vi "S4GUI_002.vi"(7 "Tab ObsEng":enum32{"Obs", "CCD modes", "Eng"}(tab)) -> ()   [LabVIEW 2018] (continued)
                n2194 = Flatten To String(anything=w4348, error in (no error)=w4351) -> (data string=w4353:string, error out=w4352:errorcluster)  [unwired: 2 in, 1 out]
                n2195 = call "Write flatted cluster.vi"("error in (no error)"=w4352, "flatted cluster"=w4353, "Interface in"=w4344) -> ("error out"=w4342:errorcluster, "Interface out"=w4343:refnum<class "Interface.lvclass">)  [unwired: 7 in]
                n2196 = call-dynamic "Write Interface.vi"("error in (no error)"=w4342, "Interface.lvclass"=w4343, "Channel in"=w4359) -> ("error out"=w4337:errorcluster, "Channel out"=w4336:refnum<class "Channel.lvclass">)  [unwired: 7 in]
                n2197 = call "Write section_name.vi"("error in (no error)"=w4337, "section_name"="CCD_ACS1", "Channel in"=w4336) -> ("error out"=w4338:errorcluster, "Channel out"=w4333:refnum<class "Channel.lvclass">)  [unwired: 7 in]
                n2198 = call-dynamic "save config.vi"("error in (no error)"=w4338, "file config"="lastsaved.cfg", "Channel in"=w4333) -> ("error out"=w4326:errorcluster, "Channel out"=w4327:refnum<class "Channel.lvclass">)  [unwired: 7 in]
                n2199 = call-dynamic "Read State Machine.vi"("error in (no error)"=w4326, "Device in"=w4327) -> ("error out"=w4341:errorcluster, "State Machine.lvclass"=w4331:refnum<class "State Machine.lvclass">, "Device out"=w4332:refnum<class "Channel.lvclass">)  [unwired: 7 in]
                n2200 = call-dynamic "Write State.vi"("error in (no error)"=w4341, "State"=60, "State Machine in"=w4331) -> ("error out"=w4340:errorcluster, "State Machine out"=w4330:refnum<class "State Machine.lvclass">)  [unwired: 7 in]
                n2201 = call-dynamic "Write State Machine.vi"("error in (no error)"=w4340, "State Machine.lvclass"=w4330, "Device in"=w4332) -> ("error out"=w4328:errorcluster, "Device out"=w4329:refnum<class "Channel.lvclass">)  [unwired: 7 in]
                n2202 = call-dynamic "Write Channel.vi"("error in (no error)"=w4328, "Channel.lvclass"=w4329, "Acquisition in"=w4358) -> ("error out"=w4355:errorcluster, "Acquisition out"=w4354:refnum<class "Acquisition.lvclass">)  [unwired: 7 in]
              }
            }
            n2203 = call-dynamic "Write AcquisitionA.vi"("error in (no error)"=w4164, "Acquisition.lvclass"=w4165, "S4ACS_GUI in"=w4166) -> ("error out"=w4172:errorcluster, "S4ACS_GUI out"=w4175:refnum<class "S4GUI.lvclass">)  [unwired: 7 in]
            n2204 = call "Write AcquisitionB.vi"("error in (no error)"=w4162, "Acquisition.lvclass"=w4163, "S4ACS_GUI in"=w4175) -> ("error out"=w4171:errorcluster, "S4ACS_GUI out"=w4174:refnum<class "S4GUI.lvclass">)  [unwired: 7 in]
            n2205 = call-dynamic "Write AcquisitionC.vi"("error in (no error)"=w4160, "Acquisition.lvclass"=w4161, "S4ACS_GUI in"=w4174) -> ("error out"=w4170:errorcluster, "S4ACS_GUI out"=w4173:refnum<class "S4GUI.lvclass">)  [unwired: 7 in]
            n2206 = call-dynamic "Write AcquisitionD.vi"("error in (no error)"=w4158, "Acquisition.lvclass"=w4159, "S4ACS_GUI in"=w4173) -> ("error out"=w4169:errorcluster, "S4ACS_GUI out"=w4168:refnum<class "S4GUI.lvclass">)  [unwired: 7 in]
            n2207 = Merge Errors(w4172, w4171, w4170, w4169) -> (w4167:errorcluster)
          }
        }
        n2208 = Concatenate Strings(w3924, " MODE SELECTED" ("User Event")) -> (w3929:string)
        n2209 = call-dynamic "Write sync.vi"("error in (no error)"=w3942, "sync"=w3944, "S4ACS_GUI in"=w3943) -> ("error out"=w3927:errorcluster, "S4ACS_GUI out"=w3928:refnum<class "S4GUI.lvclass">)  [unwired: 7 in]
        n2210 = call-dynamic "Write User Event.vi"("error in (no error)"=w3927, "User Event"=w3929, "S4GUI in"=w3928) -> ("error out"=w3925:errorcluster, "S4GUI out"=w3926:refnum<class "S4GUI.lvclass">)  [unwired: 7 in]
      }
      event "SendExpose": Value Change {
        n2211 = event-data() -> ("NewVal"=w4360:bool)  [unwired: 1 in]
        n2212 = disable-structure shown="Enabled" {
          disable-tunnel: w4360 -> [w4498 w4499]
          disable-tunnel: [w4497 w4499] -> w4361
          frame Disabled {
            n2213 = Not(x=w4498) -> (.not. x?=w4497:bool)
          }
          frame Enabled {
          }
        }
        n2214 = disable-structure shown="Enabled" {
          disable-tunnel: w4445 -> [w4460 w4496]
          disable-tunnel: w4444 -> [w4451 w4495]
          disable-tunnel: [w4448 w4496] -> w4363
          disable-tunnel: [w4447 w4495] -> w4362
          disable-tunnel: w4360 -> [w4446 _]
          frame Disabled {
            n2215 = call-dynamic "Read Sync Box.lvclass.vi"("error in (no error)"=w4451, "SPARC4_AC in"=w4460) -> ("error out"=w4453:errorcluster, "Sync Box.lvclass"=w4459:refnum<class "Sync Box.lvclass">, "SPARC4_AC out"=w4456:refnum<class "S4GUI.lvclass">)  [unwired: 7 in]
            n2216 = call-dynamic "Read Stream.vi"("error in (no error)"=w4453, "Server in"=w4459) -> ("error out"=w4452:errorcluster, "Stream.lvclass"=w4461:refnum<class "Stream.lvclass">, "Server out"=w4450:refnum<class "Sync Box.lvclass">)  [unwired: 7 in]
            n2217 = case shown="True" w4446 {
              tunnel: [w4464 w4481] -> w4454
              tunnel: w4461 -> [w4466 w4471]
              tunnel: [w4465 w4477] -> w4458
              tunnel: w4452 -> [w4463 w4469]
              tunnel: w4450 -> [w4462 w4470]
              tunnel: [w4462 w4470] -> w4449
              frame False {
                n2218 = call-dynamic "End.vi"("error in (no error)"=w4463, "Stream in"=w4466) -> ("error out"=w4464:errorcluster, "Stream out"=w4465:refnum<class "Stream.lvclass">)  [unwired: 8 in]
              }
              frame True {
                w4474 = errorcluster {"status"=FALSE, "code"=0, "source"=""} ("error in (no error)")
                w4492 = FALSE ("Wait Until Done")
                w4487 = FALSE ("Wait Until Done")
                n2219 = call-dynamic "Read comfile name1.vi"("error in (no error)"=w4469, "Stream in"=w4471) -> ("error out"=w4483:errorcluster, "comfile name1"=w4484:string, "Stream out"=w4480:refnum<class "Stream.lvclass">)  [unwired: 7 in]
                n2220 = call <vilib>:"Application Directory.vi"() -> ("Application Directory"=w4489:path)
                n2221 = call <vilib>:"Application Directory.vi"() -> ("Application Directory"=w4493:path)
                n2222 = Build Path(base path=w4493, name or relative path=w4484) -> (appended path=w4494:path)
                n2223 = Open VI Reference(vi path=w4494, error in (no error)=w4483) -> (vi reference=w4486:refnum<vi>, error out=w4485:errorcluster)  [unwired: 4 in]
                n2224 = invoke class="VI" method="Run VI"(reference=w4486, error in=w4485, "Wait until done"=w4487, "Auto Dispose Ref"=w4487) -> (reference out=w4476:refnum<vi>, error out=→"error out 7":errorcluster)  [unwired: 1 in, 3 out]
                n2225 = call-dynamic "Write commfile ref1.vi"("error in (no error)"=w4474, "commfile ref1"=w4476, "Stream in"=w4480) -> ("error out"=w4468:errorcluster, "Stream out"=w4479:refnum<class "Stream.lvclass">)  [unwired: 7 in]
                n2226 = call-dynamic "Read comfile name2.vi"("error in (no error)"=w4468, "Stream in"=w4479) -> ("error out"=w4467:errorcluster, "comfile name2"=w4482:string, "Stream out"=w4478:refnum<class "Stream.lvclass">)  [unwired: 7 in]
                n2227 = Build Path(base path=w4489, name or relative path=w4482) -> (appended path=w4488:path)
                n2228 = Open VI Reference(vi path=w4488, error in (no error)=w4467) -> (vi reference=w4490:refnum<vi>, error out=w4491:errorcluster)  [unwired: 4 in]
                n2229 = invoke class="VI" method="Run VI"(reference=w4490, error in=w4491, "Wait until done"=w4492, "Auto Dispose Ref"=w4492) -> (reference out=w4475:refnum<vi>, error out=→"error out 8":errorcluster)  [unwired: 1 in, 3 out]
                n2230 = call-dynamic "Write commfile ref2.vi"("error in (no error)"=w4474, "commfile ref2"=w4475, "Stream in"=w4478) -> ("error out"=w4481:errorcluster, "Stream out"=w4477:refnum<class "Stream.lvclass">)  [unwired: 7 in]
              }
            }
            n2231 = call-dynamic "Write Stream.vi"("error in (no error)"=w4454, "Stream.lvclass"=w4458, "Server in"=w4449) -> ("error out"=w4455:errorcluster, "Server out"=w4457:refnum<class "Sync Box.lvclass">)  [unwired: 7 in]
            n2232 = call-dynamic "Write Sync Box.lvclass.vi"("error in (no error)"=w4455, "Sync Box.lvclass"=w4457, "SPARC4_AC in"=w4456) -> ("error out"=w4447:errorcluster, "SPARC4_AC out"=w4448:refnum<class "S4GUI.lvclass">)  [unwired: 7 in]
          }
          frame Enabled {
          }
        }
        n2233 = call-dynamic "Read AcquisitionC.vi"("error in (no error)"=w4362, "S4ACS_GUI in"=w4363) -> ("error out"=w4387:errorcluster, "Acquisition.lvclass"=w4388:refnum<class "Acquisition.lvclass">)  [unwired: 7 in, 1 out]
        n2234 = call-dynamic "Read AcquisitionA.vi"("error in (no error)"=w4362, "S4ACS_GUI in"=w4363) -> ("error out"=w4424:errorcluster, "Acquisition.lvclass"=w4423:refnum<class "Acquisition.lvclass">, "S4ACS_GUI out"=w4440:refnum<class "S4GUI.lvclass">)  [unwired: 7 in]
        n2235 = call "Read AcquisitionB.vi"("error in (no error)"=w4362, "S4ACS_GUI in"=w4363) -> ("error out"=w4404:errorcluster, "Acquisition.lvclass"=w4405:refnum<class "Acquisition.lvclass">)  [unwired: 7 in, 1 out]
        n2236 = call-dynamic "Read AcquisitionD.vi"("error in (no error)"=w4362, "S4ACS_GUI in"=w4363) -> ("error out"=w4370:errorcluster, "Acquisition.lvclass"=w4371:refnum<class "Acquisition.lvclass">)  [unwired: 7 in, 1 out]
        n2237 = call-dynamic "Read Channel.vi"("error in (no error)"=w4370, "Acquisition in"=w4371) -> ("error out"=w4373:errorcluster, "Channel.lvclass"=w4375:refnum<class "Channel.lvclass">, "Acquisition out"=w4384:refnum<class "Acquisition.lvclass">)  [unwired: 7 in]
        n2238 = call-dynamic "Read Channel.vi"("error in (no error)"=w4387, "Acquisition in"=w4388) -> ("error out"=w4390:errorcluster, "Channel.lvclass"=w4392:refnum<class "Channel.lvclass">, "Acquisition out"=w4401:refnum<class "Acquisition.lvclass">)  [unwired: 7 in]
        n2239 = call-dynamic "Read Channel.vi"("error in (no error)"=w4404, "Acquisition in"=w4405) -> ("error out"=w4407:errorcluster, "Channel.lvclass"=w4409:refnum<class "Channel.lvclass">, "Acquisition out"=w4418:refnum<class "Acquisition.lvclass">)  [unwired: 7 in]
        n2240 = call-dynamic "Read Channel.vi"("error in (no error)"=w4424, "Acquisition in"=w4423) -> ("error out"=w4420:errorcluster, "Channel.lvclass"=w4422:refnum<class "Channel.lvclass">, "Acquisition out"=w4433:refnum<class "Acquisition.lvclass">)  [unwired: 7 in]
        n2241 = call-dynamic "Write wait_expose.vi"("error in (no error)"=w4373, "wait_expose"=w4361, "Channel in"=w4375) -> ("error out"=w4372:errorcluster, "Channel out"=w4374:refnum<class "Channel.lvclass">)  [unwired: 7 in]
        n2242 = call-dynamic "Write wait_expose.vi"("error in (no error)"=w4390, "wait_expose"=w4361, "Channel in"=w4392) -> ("error out"=w4389:errorcluster, "Channel out"=w4391:refnum<class "Channel.lvclass">)  [unwired: 7 in]
        n2243 = call-dynamic "Write wait_expose.vi"("error in (no error)"=w4407, "wait_expose"=w4361, "Channel in"=w4409) -> ("error out"=w4406:errorcluster, "Channel out"=w4408:refnum<class "Channel.lvclass">)  [unwired: 7 in]
        n2244 = call-dynamic "Write wait_expose.vi"("error in (no error)"=w4420, "wait_expose"=w4361, "Channel in"=w4422) -> ("error out"=w4419:errorcluster, "Channel out"=w4421:refnum<class "Channel.lvclass">)  [unwired: 7 in]
        n2245 = call-dynamic "Read State Machine.vi"("error in (no error)"=w4372, "Device in"=w4374) -> ("error out"=w4383:errorcluster, "State Machine.lvclass"=w4379:refnum<class "State Machine.lvclass">, "Device out"=w4380:refnum<class "Channel.lvclass">)  [unwired: 7 in]
        n2246 = call-dynamic "Read State Machine.vi"("error in (no error)"=w4389, "Device in"=w4391) -> ("error out"=w4400:errorcluster, "State Machine.lvclass"=w4396:refnum<class "State Machine.lvclass">, "Device out"=w4397:refnum<class "Channel.lvclass">)  [unwired: 7 in]
        n2247 = call-dynamic "Read State Machine.vi"("error in (no error)"=w4406, "Device in"=w4408) -> ("error out"=w4417:errorcluster, "State Machine.lvclass"=w4413:refnum<class "State Machine.lvclass">, "Device out"=w4414:refnum<class "Channel.lvclass">)  [unwired: 7 in]
        n2248 = call-dynamic "Read State Machine.vi"("error in (no error)"=w4419, "Device in"=w4421) -> ("error out"=w4432:errorcluster, "State Machine.lvclass"=w4428:refnum<class "State Machine.lvclass">, "Device out"=w4429:refnum<class "Channel.lvclass">)  [unwired: 7 in]
        n2249 = call-dynamic "Write State.vi"("error in (no error)"=w4383, "State"=40, "State Machine in"=w4379) -> ("error out"=w4382:errorcluster, "State Machine out"=w4378:refnum<class "State Machine.lvclass">)  [unwired: 7 in]
        n2250 = call-dynamic "Write State.vi"("error in (no error)"=w4400, "State"=40, "State Machine in"=w4396) -> ("error out"=w4399:errorcluster, "State Machine out"=w4395:refnum<class "State Machine.lvclass">)  [unwired: 7 in]
        n2251 = call-dynamic "Write State.vi"("error in (no error)"=w4417, "State"=40, "State Machine in"=w4413) -> ("error out"=w4416:errorcluster, "State Machine out"=w4412:refnum<class "State Machine.lvclass">)  [unwired: 7 in]
        n2252 = call-dynamic "Write State.vi"("error in (no error)"=w4432, "State"=40, "State Machine in"=w4428) -> ("error out"=w4431:errorcluster, "State Machine out"=w4427:refnum<class "State Machine.lvclass">)  [unwired: 7 in]
        n2253 = call-dynamic "Write State Machine.vi"("error in (no error)"=w4382, "State Machine.lvclass"=w4378, "Device in"=w4380) -> ("error out"=w4376:errorcluster, "Device out"=w4377:refnum<class "Channel.lvclass">)  [unwired: 7 in]
        n2254 = call-dynamic "Write State Machine.vi"("error in (no error)"=w4399, "State Machine.lvclass"=w4395, "Device in"=w4397) -> ("error out"=w4393:errorcluster, "Device out"=w4394:refnum<class "Channel.lvclass">)  [unwired: 7 in]
        n2255 = call-dynamic "Write State Machine.vi"("error in (no error)"=w4416, "State Machine.lvclass"=w4412, "Device in"=w4414) -> ("error out"=w4410:errorcluster, "Device out"=w4411:refnum<class "Channel.lvclass">)  [unwired: 7 in]
        n2256 = call-dynamic "Write State Machine.vi"("error in (no error)"=w4431, "State Machine.lvclass"=w4427, "Device in"=w4429) -> ("error out"=w4425:errorcluster, "Device out"=w4426:refnum<class "Channel.lvclass">)  [unwired: 7 in]
        n2257 = call-dynamic "Write Channel.vi"("error in (no error)"=w4376, "Channel.lvclass"=w4377, "Acquisition in"=w4384) -> ("error out"=w4368:errorcluster, "Acquisition out"=w4369:refnum<class "Acquisition.lvclass">)  [unwired: 7 in]
        n2258 = call-dynamic "Write Channel.vi"("error in (no error)"=w4393, "Channel.lvclass"=w4394, "Acquisition in"=w4401) -> ("error out"=w4386:errorcluster, "Acquisition out"=w4385:refnum<class "Acquisition.lvclass">)  [unwired: 7 in]
        n2259 = call-dynamic "Write Channel.vi"("error in (no error)"=w4410, "Channel.lvclass"=w4411, "Acquisition in"=w4418) -> ("error out"=w4403:errorcluster, "Acquisition out"=w4402:refnum<class "Acquisition.lvclass">)  [unwired: 7 in]
        n2260 = call-dynamic "Write Channel.vi"("error in (no error)"=w4425, "Channel.lvclass"=w4426, "Acquisition in"=w4433) -> ("error out"=w4438:errorcluster, "Acquisition out"=w4439:refnum<class "Acquisition.lvclass">)  [unwired: 7 in]
        n2261 = call-dynamic "Write AcquisitionA.vi"("error in (no error)"=w4438, "Acquisition.lvclass"=w4439, "S4ACS_GUI in"=w4440) -> ("error out"=w4437:errorcluster, "S4ACS_GUI out"=w4443:refnum<class "S4GUI.lvclass">)  [unwired: 7 in]
        n2262 = call "Write AcquisitionB.vi"("error in (no error)"=w4403, "Acquisition.lvclass"=w4402, "S4ACS_GUI in"=w4443) -> ("error out"=w4436:errorcluster, "S4ACS_GUI out"=w4442:refnum<class "S4GUI.lvclass">)  [unwired: 7 in]
        n2263 = call-dynamic "Write AcquisitionC.vi"("error in (no error)"=w4386, "Acquisition.lvclass"=w4385, "S4ACS_GUI in"=w4442) -> ("error out"=w4435:errorcluster, "S4ACS_GUI out"=w4441:refnum<class "S4GUI.lvclass">)  [unwired: 7 in]
        n2264 = call-dynamic "Write AcquisitionD.vi"("error in (no error)"=w4368, "Acquisition.lvclass"=w4369, "S4ACS_GUI in"=w4441) -> ("error out"=w4434:errorcluster, "S4ACS_GUI out"=w4367:refnum<class "S4GUI.lvclass">)  [unwired: 7 in]
        n2265 = Merge Errors(w4437, w4436, w4435, w4434) -> (w4366:errorcluster)
        n2266 = call-dynamic "Write mode EXPOSE.vi"("error in (no error)"=w4366, "mode EXPOSE"=w4361, "S4GUI in"=w4367) -> ("error out"=w4364:errorcluster, "S4GUI out"=w4365:refnum<class "S4GUI.lvclass">)  [unwired: 7 in]
      }
      event "CH1on": Value Change {
        n2267 = event-data() -> ("NewVal"=w4509:bool)  [unwired: 1 in]
        n2268 = call-dynamic "Read AcquisitionA.vi"("error in (no error)"=w4523, "S4ACS_GUI in"=w4524) -> ("error out"=w4515:errorcluster, "Acquisition.lvclass"=w4520:refnum<class "Acquisition.lvclass">, "S4ACS_GUI out"=w4516:refnum<class "S4GUI.lvclass">)  [unwired: 7 in]
        n2269 = call-dynamic "Read Channel.vi"("error in (no error)"=w4515, "Acquisition in"=w4520) -> ("error out"=w4514:errorcluster, "Channel.lvclass"=w4505:refnum<class "Channel.lvclass">, "Acquisition out"=w4519:refnum<class "Acquisition.lvclass">)  [unwired: 7 in]
        n2270 = call-dynamic "Read Stream.vi"("error in (no error)"=w4514, "Server in"=w4519) -> ("error out"=w4507:errorcluster, "Stream.lvclass"=w4508:refnum<class "Stream.lvclass">, "Server out"=w4506:refnum<class "Acquisition.lvclass">)  [unwired: 7 in]
        n2271 = case shown="False" w4509 {
          selector: w4509 -> [w4525 w4547]
          tunnel: [w4531 w4551] -> w4503
          tunnel: w4508 -> [w4540 _]
          tunnel: [w4539 w4554] -> w4502
          tunnel: w4507 -> [w4526 w4548]
          tunnel: w4506 -> [w4527 w4549]
          tunnel: [w4527 w4553] -> w4501
          tunnel: w4505 -> [w4538 w4550]
          tunnel: [w4536 w4550] -> w4500
          tunnel: [w4525 w4547] -> w4504
          frame False {
            # "força FALSE nos parametros do CCD"
            n2272 = call-dynamic "Read Interface.vi"("error in (no error)"=w4526, "Channel in"=w4538) -> ("error out"=w4535:errorcluster, "Interface.lvclass"=w4529:refnum<class "Interface.lvclass">, "Channel out"=w4537:refnum<class "Channel.lvclass">)  [unwired: 7 in]
            n2273 = disable-structure shown="Enabled" {
              disable-tunnel: w4540 -> [w4544 w4546]
              disable-tunnel: [w4543 w4546] -> w4539
              disable-tunnel: [w4542 w4545] -> w4532
              disable-tunnel: w4526 -> [w4541 w4545]
              frame Disabled {
                n2274 = call-dynamic "End.vi"("error in (no error)"=w4541, "Stream in"=w4544) -> ("error out"=w4542:errorcluster, "Stream out"=w4543:refnum<class "Stream.lvclass">)  [unwired: 8 in]
              }
              frame Enabled {
              }
            }
            n2275 = call "Write Checked Params.vi"("error in (no error)"=w4535, "Checked Params"=T14 {"ACQUISITION_MODE"=FALSE, "TRIGGER_MODE"=FALSE, "READ_MODE"=FALSE, "PREAMP"=FALSE, "READOUT_RATE"=FALSE, "VERTICAL_SHIFT_SPEED"=FALSE, "EM_MODE"=FALSE, "EM_GAIN"=FALSE, "SHUTTER_MODE"=FALSE, "SHUTTER_TTL"=FALSE, "SHUTTER_OPENING_TIME"=FALSE, "SHUTTER_CLOSING_TIME"=FALSE, "VBIN"=FALSE, "HBIN"=FALSE, "INITIAL_LINE"=FALSE, "INITIAL_COLUMN"=FALSE, "FINAL_LINE"=FALSE, "FINAL_COLUMN"=FALSE, "FRAME_TRANSFER"=FALSE, "VERTICAL_CLOCK_VOLTAGE"=FALSE, "AD_CHANNEL"=FALSE}, "Interface in"=w4529) -> ("error out"=w4534:errorcluster, "Interface out"=w4528:refnum<class "Interface.lvclass">)  [unwired: 7 in]
            n2276 = call-dynamic "Write Interface.vi"("error in (no error)"=w4534, "Interface.lvclass"=w4528, "Channel in"=w4537) -> ("error out"=w4533:errorcluster, "Channel out"=w4536:refnum<class "Channel.lvclass">)  [unwired: 7 in]
            n2277 = Merge Errors(w4533, w4532) -> (w4531:errorcluster)
          }
          frame True {
            n2278 = call-dynamic "Read Stream.vi"("error in (no error)"=w4548, "Server in"=w4549) -> ("error out"=w4552:errorcluster, "Stream.lvclass"=w4555:refnum<class "Stream.lvclass">, "Server out"=w4553:refnum<class "Acquisition.lvclass">)  [unwired: 7 in]
            n2279 = disable-structure shown="Enabled" {
              disable-tunnel: w4555 -> [w4561 w4571]
              disable-tunnel: [w4560 w4571] -> w4554
              disable-tunnel: w4552 -> [w4558 w4570]
              disable-tunnel: [w4556 w4570] -> w4551
              frame Disabled {
                w4569 = FALSE ("Wait Until Done")
                n2280 = call-dynamic "Read comfile name1.vi"("error in (no error)"=w4558, "Stream in"=w4561) -> ("error out"=w4557:errorcluster, "comfile name1"=w4564:string, "Stream out"=w4559:refnum<class "Stream.lvclass">)  [unwired: 7 in]
                n2281 = call <vilib>:"Application Directory.vi"() -> ("Application Directory"=w4566:path)
                n2282 = Build Path(base path=w4566, name or relative path=w4564) -> (appended path=w4565:path)
                n2283 = Open VI Reference(vi path=w4565, error in (no error)=w4557) -> (vi reference=w4567:refnum<vi>, error out=w4568:errorcluster)  [unwired: 4 in]
                n2284 = invoke class="VI" method="Run VI"(reference=w4567, error in=w4568, "Wait until done"=w4569, "Auto Dispose Ref"=w4569) -> (reference out=w4563:refnum<vi>, error out=w4562:errorcluster)  [unwired: 1 in, 3 out]
                n2285 = call-dynamic "Write commfile ref1.vi"("error in (no error)"=w4562, "commfile ref1"=w4563, "Stream in"=w4559) -> ("error out"=w4556:errorcluster, "Stream out"=w4560:refnum<class "Stream.lvclass">)  [unwired: 7 in]
              }
              frame Enabled {
              }
            }
          }
        }
        n2286 = call-dynamic "Write Stream.vi"("error in (no error)"=w4503, "Stream.lvclass"=w4502, "Server in"=w4501) -> ("error out"=w4513:errorcluster, "Server out"=w4511:refnum<class "Acquisition.lvclass">)  [unwired: 7 in]
        n2287 = call-dynamic "Write enabled.vi"("error in (no error)"=w4513, "enabled"=w4504, "Server in"=w4511) -> ("error out"=w4512:errorcluster, "Server out"=w4510:refnum<class "Acquisition.lvclass">)  [unwired: 7 in]
        n2288 = call-dynamic "Write Channel.vi"("error in (no error)"=w4512, "Channel.lvclass"=w4500, "Acquisition in"=w4510) -> ("error out"=w4518:errorcluster, "Acquisition out"=w4517:refnum<class "Acquisition.lvclass">)  [unwired: 7 in]
        n2289 = call-dynamic "Write AcquisitionA.vi"("error in (no error)"=w4518, "Acquisition.lvclass"=w4517, "S4ACS_GUI in"=w4516) -> ("error out"=w4521:errorcluster, "S4ACS_GUI out"=w4522:refnum<class "S4GUI.lvclass">)  [unwired: 7 in]
      }
      event "CH2on": Value Change {
        n2290 = event-data() -> ("NewVal"=w4573:bool)  [unwired: 1 in]
        n2291 = call "Read AcquisitionB.vi"("error in (no error)"=w4595, "S4ACS_GUI in"=w4596) -> ("error out"=w4587:errorcluster, "Acquisition.lvclass"=w4592:refnum<class "Acquisition.lvclass">, "S4ACS_GUI out"=w4588:refnum<class "S4GUI.lvclass">)  [unwired: 7 in]
        n2292 = call-dynamic "Read Channel.vi"("error in (no error)"=w4587, "Acquisition in"=w4592) -> ("error out"=w4586:errorcluster, "Channel.lvclass"=w4581:refnum<class "Channel.lvclass">, "Acquisition out"=w4591:refnum<class "Acquisition.lvclass">)  [unwired: 7 in]
        n2293 = call-dynamic "Read Stream.vi"("error in (no error)"=w4586, "Server in"=w4591) -> ("error out"=w4577:errorcluster, "Stream.lvclass"=w4574:refnum<class "Stream.lvclass">, "Server out"=w4579:refnum<class "Acquisition.lvclass">)  [unwired: 7 in]
        n2294 = case shown="False" w4573 {
          selector: w4573 -> [w4597 w4619]
          tunnel: [w4603 w4623] -> w4576
          tunnel: w4574 -> [w4612 _]
          tunnel: [w4611 w4626] -> w4575
          tunnel: w4577 -> [w4598 w4620]
          tunnel: w4579 -> [w4599 w4621]
          tunnel: [w4599 w4625] -> w4578
          tunnel: w4581 -> [w4610 w4622]
          tunnel: [w4608 w4622] -> w4580
          tunnel: [w4597 w4619] -> w4572
          frame False {
            # "força FALSE nos parametros do CCD"
            n2295 = call-dynamic "Read Interface.vi"("error in (no error)"=w4598, "Channel in"=w4610) -> ("error out"=w4607:errorcluster, "Interface.lvclass"=w4601:refnum<class "Interface.lvclass">, "Channel out"=w4609:refnum<class "Channel.lvclass">)  [unwired: 7 in]
            n2296 = disable-structure shown="Enabled" {
              disable-tunnel: w4612 -> [w4616 w4618]
              disable-tunnel: [w4615 w4618] -> w4611
              disable-tunnel: [w4614 w4617] -> w4604
              disable-tunnel: w4598 -> [w4613 w4617]
              frame Disabled {
                n2297 = call-dynamic "End.vi"("error in (no error)"=w4613, "Stream in"=w4616) -> ("error out"=w4614:errorcluster, "Stream out"=w4615:refnum<class "Stream.lvclass">)  [unwired: 8 in]
              }
              frame Enabled {
              }
            }
            n2298 = call "Write Checked Params.vi"("error in (no error)"=w4607, "Checked Params"=T14 {"ACQUISITION_MODE"=FALSE, "TRIGGER_MODE"=FALSE, "READ_MODE"=FALSE, "PREAMP"=FALSE, "READOUT_RATE"=FALSE, "VERTICAL_SHIFT_SPEED"=FALSE, "EM_MODE"=FALSE, "EM_GAIN"=FALSE, "SHUTTER_MODE"=FALSE, "SHUTTER_TTL"=FALSE, "SHUTTER_OPENING_TIME"=FALSE, "SHUTTER_CLOSING_TIME"=FALSE, "VBIN"=FALSE, "HBIN"=FALSE, "INITIAL_LINE"=FALSE, "INITIAL_COLUMN"=FALSE, "FINAL_LINE"=FALSE, "FINAL_COLUMN"=FALSE, "FRAME_TRANSFER"=FALSE, "VERTICAL_CLOCK_VOLTAGE"=FALSE, "AD_CHANNEL"=FALSE}, "Interface in"=w4601) -> ("error out"=w4606:errorcluster, "Interface out"=w4600:refnum<class "Interface.lvclass">)  [unwired: 7 in]
            n2299 = call-dynamic "Write Interface.vi"("error in (no error)"=w4606, "Interface.lvclass"=w4600, "Channel in"=w4609) -> ("error out"=w4605:errorcluster, "Channel out"=w4608:refnum<class "Channel.lvclass">)  [unwired: 7 in]
            n2300 = Merge Errors(w4605, w4604) -> (w4603:errorcluster)
          }
          frame True {
            n2301 = call-dynamic "Read Stream.vi"("error in (no error)"=w4620, "Server in"=w4621) -> ("error out"=w4624:errorcluster, "Stream.lvclass"=w4627:refnum<class "Stream.lvclass">, "Server out"=w4625:refnum<class "Acquisition.lvclass">)  [unwired: 7 in]
            n2302 = disable-structure shown="Enabled" {
              disable-tunnel: w4627 -> [w4633 w4643]
              disable-tunnel: [w4632 w4643] -> w4626
              disable-tunnel: w4624 -> [w4630 w4642]
              disable-tunnel: [w4628 w4642] -> w4623
              frame Disabled {
                w4641 = FALSE ("Wait Until Done")
                n2303 = call-dynamic "Read comfile name1.vi"("error in (no error)"=w4630, "Stream in"=w4633) -> ("error out"=w4629:errorcluster, "comfile name1"=w4636:string, "Stream out"=w4631:refnum<class "Stream.lvclass">)  [unwired: 7 in]
                n2304 = call <vilib>:"Application Directory.vi"() -> ("Application Directory"=w4638:path)
                n2305 = Build Path(base path=w4638, name or relative path=w4636) -> (appended path=w4637:path)
                n2306 = Open VI Reference(vi path=w4637, error in (no error)=w4629) -> (vi reference=w4639:refnum<vi>, error out=w4640:errorcluster)  [unwired: 4 in]
                n2307 = invoke class="VI" method="Run VI"(reference=w4639, error in=w4640, "Wait until done"=w4641, "Auto Dispose Ref"=w4641) -> (reference out=w4635:refnum<vi>, error out=w4634:errorcluster)  [unwired: 1 in, 3 out]
                n2308 = call-dynamic "Write commfile ref1.vi"("error in (no error)"=w4634, "commfile ref1"=w4635, "Stream in"=w4631) -> ("error out"=w4628:errorcluster, "Stream out"=w4632:refnum<class "Stream.lvclass">)  [unwired: 7 in]
              }
              frame Enabled {
              }
            }
          }
        }
        n2309 = call-dynamic "Write Stream.vi"("error in (no error)"=w4576, "Stream.lvclass"=w4575, "Server in"=w4578) -> ("error out"=w4583:errorcluster, "Server out"=w4585:refnum<class "Acquisition.lvclass">)  [unwired: 7 in]
        n2310 = call-dynamic "Write enabled.vi"("error in (no error)"=w4583, "enabled"=w4572, "Server in"=w4585) -> ("error out"=w4582:errorcluster, "Server out"=w4584:refnum<class "Acquisition.lvclass">)  [unwired: 7 in]
        n2311 = call-dynamic "Write Channel.vi"("error in (no error)"=w4582, "Channel.lvclass"=w4580, "Acquisition in"=w4584) -> ("error out"=w4590:errorcluster, "Acquisition out"=w4589:refnum<class "Acquisition.lvclass">)  [unwired: 7 in]
        n2312 = call "Write AcquisitionB.vi"("error in (no error)"=w4590, "Acquisition.lvclass"=w4589, "S4ACS_GUI in"=w4588) -> ("error out"=w4593:errorcluster, "S4ACS_GUI out"=w4594:refnum<class "S4GUI.lvclass">)  [unwired: 7 in]
      }
      event "CH3 on": Value Change {
        n2313 = event-data() -> ("NewVal"=w4660:bool)  [unwired: 1 in]
        n2314 = call-dynamic "Read AcquisitionC.vi"("error in (no error)"=w4663, "S4ACS_GUI in"=w4667) -> ("error out"=w4652:errorcluster, "Acquisition.lvclass"=w4657:refnum<class "Acquisition.lvclass">, "S4ACS_GUI out"=w4653:refnum<class "S4GUI.lvclass">)  [unwired: 7 in]
        n2315 = call-dynamic "Read Channel.vi"("error in (no error)"=w4652, "Acquisition in"=w4657) -> ("error out"=w4651:errorcluster, "Channel.lvclass"=w4650:refnum<class "Channel.lvclass">, "Acquisition out"=w4656:refnum<class "Acquisition.lvclass">)  [unwired: 7 in]
        n2316 = call-dynamic "Read Stream.vi"("error in (no error)"=w4651, "Server in"=w4656) -> ("error out"=w4664:errorcluster, "Stream.lvclass"=w4668:refnum<class "Stream.lvclass">, "Server out"=w4662:refnum<class "Acquisition.lvclass">)  [unwired: 7 in]
        n2317 = case shown="False" w4660 {
          selector: w4660 -> [w4669 w4691]
          tunnel: [w4675 w4695] -> w4665
          tunnel: w4668 -> [w4684 _]
          tunnel: [w4683 w4698] -> w4666
          tunnel: w4664 -> [w4670 w4692]
          tunnel: w4662 -> [w4671 w4693]
          tunnel: [w4671 w4697] -> w4661
          tunnel: w4650 -> [w4682 w4694]
          tunnel: [w4680 w4694] -> w4649
          tunnel: [w4669 w4691] -> w4644
          frame False {
            # "força FALSE nos parametros do CCD"
            n2318 = call-dynamic "Read Interface.vi"("error in (no error)"=w4670, "Channel in"=w4682) -> ("error out"=w4679:errorcluster, "Interface.lvclass"=w4673:refnum<class "Interface.lvclass">, "Channel out"=w4681:refnum<class "Channel.lvclass">)  [unwired: 7 in]
            n2319 = disable-structure shown="Disabled" {
              disable-tunnel: w4684 -> [w4688 w4690]
              disable-tunnel: [w4687 w4690] -> w4683
              disable-tunnel: [w4686 w4689] -> w4676
              disable-tunnel: w4670 -> [w4685 w4689]
              frame Disabled {
                n2320 = call-dynamic "End.vi"("error in (no error)"=w4685, "Stream in"=w4688) -> ("error out"=w4686:errorcluster, "Stream out"=w4687:refnum<class "Stream.lvclass">)  [unwired: 8 in]
              }
              frame Enabled {
              }
            }
            n2321 = call "Write Checked Params.vi"("error in (no error)"=w4679, "Checked Params"=T14 {"ACQUISITION_MODE"=FALSE, "TRIGGER_MODE"=FALSE, "READ_MODE"=FALSE, "PREAMP"=FALSE, "READOUT_RATE"=FALSE, "VERTICAL_SHIFT_SPEED"=FALSE, "EM_MODE"=FALSE, "EM_GAIN"=FALSE, "SHUTTER_MODE"=FALSE, "SHUTTER_TTL"=FALSE, "SHUTTER_OPENING_TIME"=FALSE, "SHUTTER_CLOSING_TIME"=FALSE, "VBIN"=FALSE, "HBIN"=FALSE, "INITIAL_LINE"=FALSE, "INITIAL_COLUMN"=FALSE, "FINAL_LINE"=FALSE, "FINAL_COLUMN"=FALSE, "FRAME_TRANSFER"=FALSE, "VERTICAL_CLOCK_VOLTAGE"=FALSE, "AD_CHANNEL"=FALSE}, "Interface in"=w4673) -> ("error out"=w4678:errorcluster, "Interface out"=w4672:refnum<class "Interface.lvclass">)  [unwired: 7 in]
            n2322 = call-dynamic "Write Interface.vi"("error in (no error)"=w4678, "Interface.lvclass"=w4672, "Channel in"=w4681) -> ("error out"=w4677:errorcluster, "Channel out"=w4680:refnum<class "Channel.lvclass">)  [unwired: 7 in]
            n2323 = Merge Errors(w4677, w4676) -> (w4675:errorcluster)
          }
          frame True {
            n2324 = call-dynamic "Read Stream.vi"("error in (no error)"=w4692, "Server in"=w4693) -> ("error out"=w4696:errorcluster, "Stream.lvclass"=w4699:refnum<class "Stream.lvclass">, "Server out"=w4697:refnum<class "Acquisition.lvclass">)  [unwired: 7 in]
            n2325 = disable-structure shown="Enabled" {
              disable-tunnel: w4699 -> [w4705 w4715]
              disable-tunnel: [w4704 w4715] -> w4698
              disable-tunnel: w4696 -> [w4702 w4714]
              disable-tunnel: [w4700 w4714] -> w4695
              frame Disabled {
                w4713 = FALSE ("Wait Until Done")
                n2326 = call-dynamic "Read comfile name1.vi"("error in (no error)"=w4702, "Stream in"=w4705) -> ("error out"=w4701:errorcluster, "comfile name1"=w4708:string, "Stream out"=w4703:refnum<class "Stream.lvclass">)  [unwired: 7 in]
                n2327 = call <vilib>:"Application Directory.vi"() -> ("Application Directory"=w4710:path)
                n2328 = Build Path(base path=w4710, name or relative path=w4708) -> (appended path=w4709:path)
                n2329 = Open VI Reference(vi path=w4709, error in (no error)=w4701) -> (vi reference=w4711:refnum<vi>, error out=w4712:errorcluster)  [unwired: 4 in]
                n2330 = invoke class="VI" method="Run VI"(reference=w4711, error in=w4712, "Wait until done"=w4713, "Auto Dispose Ref"=w4713) -> (reference out=w4707:refnum<vi>, error out=w4706:errorcluster)  [unwired: 1 in, 3 out]
                n2331 = call-dynamic "Write commfile ref1.vi"("error in (no error)"=w4706, "commfile ref1"=w4707, "Stream in"=w4703) -> ("error out"=w4700:errorcluster, "Stream out"=w4704:refnum<class "Stream.lvclass">)  [unwired: 7 in]
              }
              frame Enabled {
              }
            }
          }
        }
        n2332 = call-dynamic "Write Stream.vi"("error in (no error)"=w4665, "Stream.lvclass"=w4666, "Server in"=w4661) -> ("error out"=w4647:errorcluster, "Server out"=w4648:refnum<class "Acquisition.lvclass">)  [unwired: 7 in]
        n2333 = call-dynamic "Write enabled.vi"("error in (no error)"=w4647, "enabled"=w4644, "Server in"=w4648) -> ("error out"=w4645:errorcluster, "Server out"=w4646:refnum<class "Acquisition.lvclass">)  [unwired: 7 in]
        n2334 = call-dynamic "Write Channel.vi"("error in (no error)"=w4645, "Channel.lvclass"=w4649, "Acquisition in"=w4646) -> ("error out"=w4655:errorcluster, "Acquisition out"=w4654:refnum<class "Acquisition.lvclass">)  [unwired: 7 in]
        n2335 = call-dynamic "Write AcquisitionC.vi"("error in (no error)"=w4655, "Acquisition.lvclass"=w4654, "S4ACS_GUI in"=w4653) -> ("error out"=w4658:errorcluster, "S4ACS_GUI out"=w4659:refnum<class "S4GUI.lvclass">)  [unwired: 7 in]
      }
      event "CH4 on": Value Change {
        n2336 = event-data() -> ("NewVal"=w4721:bool)  [unwired: 1 in]
        n2337 = call-dynamic "Read AcquisitionD.vi"("error in (no error)"=w4739, "S4ACS_GUI in"=w4740) -> ("error out"=w4731:errorcluster, "Acquisition.lvclass"=w4736:refnum<class "Acquisition.lvclass">, "S4ACS_GUI out"=w4732:refnum<class "S4GUI.lvclass">)  [unwired: 7 in]
        n2338 = call-dynamic "Read Channel.vi"("error in (no error)"=w4731, "Acquisition in"=w4736) -> ("error out"=w4730:errorcluster, "Channel.lvclass"=w4725:refnum<class "Channel.lvclass">, "Acquisition out"=w4735:refnum<class "Acquisition.lvclass">)  [unwired: 7 in]
        n2339 = call-dynamic "Read Stream.vi"("error in (no error)"=w4730, "Server in"=w4735) -> ("error out"=w4723:errorcluster, "Stream.lvclass"=w4722:refnum<class "Stream.lvclass">, "Server out"=w4724:refnum<class "Acquisition.lvclass">)  [unwired: 7 in]
        n2340 = case shown="False" w4721 {
          selector: w4721 -> [w4741 w4763]
          tunnel: [w4747 w4767] -> w4717
          tunnel: w4722 -> [w4756 _]
          tunnel: [w4755 w4770] -> w4718
          tunnel: w4723 -> [w4742 w4764]
          tunnel: w4724 -> [w4743 w4765]
          tunnel: [w4743 w4769] -> w4719
          tunnel: w4725 -> [w4754 w4766]
          tunnel: [w4752 w4766] -> w4720
          tunnel: [w4741 w4763] -> w4716
          frame False {
            # "força FALSE nos parametros do CCD"
            n2341 = call-dynamic "Read Interface.vi"("error in (no error)"=w4742, "Channel in"=w4754) -> ("error out"=w4751:errorcluster, "Interface.lvclass"=w4745:refnum<class "Interface.lvclass">, "Channel out"=w4753:refnum<class "Channel.lvclass">)  [unwired: 7 in]
            n2342 = disable-structure shown="Disabled" {
              disable-tunnel: w4756 -> [w4760 w4762]
              disable-tunnel: [w4759 w4762] -> w4755
              disable-tunnel: [w4758 w4761] -> w4748
              disable-tunnel: w4742 -> [w4757 w4761]
              frame Disabled {
                n2343 = call-dynamic "End.vi"("error in (no error)"=w4757, "Stream in"=w4760) -> ("error out"=w4758:errorcluster, "Stream out"=w4759:refnum<class "Stream.lvclass">)  [unwired: 8 in]
              }
              frame Enabled {
              }
            }
            n2344 = call "Write Checked Params.vi"("error in (no error)"=w4751, "Checked Params"=T14 {"ACQUISITION_MODE"=FALSE, "TRIGGER_MODE"=FALSE, "READ_MODE"=FALSE, "PREAMP"=FALSE, "READOUT_RATE"=FALSE, "VERTICAL_SHIFT_SPEED"=FALSE, "EM_MODE"=FALSE, "EM_GAIN"=FALSE, "SHUTTER_MODE"=FALSE, "SHUTTER_TTL"=FALSE, "SHUTTER_OPENING_TIME"=FALSE, "SHUTTER_CLOSING_TIME"=FALSE, "VBIN"=FALSE, "HBIN"=FALSE, "INITIAL_LINE"=FALSE, "INITIAL_COLUMN"=FALSE, "FINAL_LINE"=FALSE, "FINAL_COLUMN"=FALSE, "FRAME_TRANSFER"=FALSE, "VERTICAL_CLOCK_VOLTAGE"=FALSE, "AD_CHANNEL"=FALSE}, "Interface in"=w4745) -> ("error out"=w4750:errorcluster, "Interface out"=w4744:refnum<class "Interface.lvclass">)  [unwired: 7 in]
            n2345 = call-dynamic "Write Interface.vi"("error in (no error)"=w4750, "Interface.lvclass"=w4744, "Channel in"=w4753) -> ("error out"=w4749:errorcluster, "Channel out"=w4752:refnum<class "Channel.lvclass">)  [unwired: 7 in]
            n2346 = Merge Errors(w4749, w4748) -> (w4747:errorcluster)
          }
          frame True {
            n2347 = call-dynamic "Read Stream.vi"("error in (no error)"=w4764, "Server in"=w4765) -> ("error out"=w4768:errorcluster, "Stream.lvclass"=w4771:refnum<class "Stream.lvclass">, "Server out"=w4769:refnum<class "Acquisition.lvclass">)  [unwired: 7 in]
            n2348 = disable-structure shown="Enabled" {
              disable-tunnel: w4771 -> [w4777 w4787]
              disable-tunnel: [w4776 w4787] -> w4770
              disable-tunnel: w4768 -> [w4774 w4786]
              disable-tunnel: [w4772 w4786] -> w4767
              frame Disabled {
                w4785 = FALSE ("Wait Until Done")
                n2349 = call-dynamic "Read comfile name1.vi"("error in (no error)"=w4774, "Stream in"=w4777) -> ("error out"=w4773:errorcluster, "comfile name1"=w4780:string, "Stream out"=w4775:refnum<class "Stream.lvclass">)  [unwired: 7 in]
                n2350 = call <vilib>:"Application Directory.vi"() -> ("Application Directory"=w4782:path)
                n2351 = Build Path(base path=w4782, name or relative path=w4780) -> (appended path=w4781:path)
                n2352 = Open VI Reference(vi path=w4781, error in (no error)=w4773) -> (vi reference=w4783:refnum<vi>, error out=w4784:errorcluster)  [unwired: 4 in]
                n2353 = invoke class="VI" method="Run VI"(reference=w4783, error in=w4784, "Wait until done"=w4785, "Auto Dispose Ref"=w4785) -> (reference out=w4779:refnum<vi>, error out=w4778:errorcluster)  [unwired: 1 in, 3 out]
                n2354 = call-dynamic "Write commfile ref1.vi"("error in (no error)"=w4778, "commfile ref1"=w4779, "Stream in"=w4775) -> ("error out"=w4772:errorcluster, "Stream out"=w4776:refnum<class "Stream.lvclass">)  [unwired: 7 in]
              }
              frame Enabled {
              }
            }
          }
        }
        n2355 = call-dynamic "Write Stream.vi"("error in (no error)"=w4717, "Stream.lvclass"=w4718, "Server in"=w4719) -> ("error out"=w4727:errorcluster, "Server out"=w4729:refnum<class "Acquisition.lvclass">)  [unwired: 7 in]
        n2356 = call-dynamic "Write enabled.vi"("error in (no error)"=w4727, "enabled"=w4716, "Server in"=w4729) -> ("error out"=w4726:errorcluster, "Server out"=w4728:refnum<class "Acquisition.lvclass">)  [unwired: 7 in]
        n2357 = call-dynamic "Write Channel.vi"("error in (no error)"=w4726, "Channel.lvclass"=w4720, "Acquisition in"=w4728) -> ("error out"=w4734:errorcluster, "Acquisition out"=w4733:refnum<class "Acquisition.lvclass">)  [unwired: 7 in]
        n2358 = call-dynamic "Write AcquisitionD.vi"("error in (no error)"=w4734, "Acquisition.lvclass"=w4733, "S4ACS_GUI in"=w4732) -> ("error out"=w4737:errorcluster, "S4ACS_GUI out"=w4738:refnum<class "S4GUI.lvclass">)  [unwired: 7 in]
      }
      event "Run WPROT": Value Change {
        n2359 = event-data() -> ("NewVal"=w4795:bool)  [unwired: 1 in]
        n2360 = case shown="True" w4795 {
          tunnel: [u32 0 ("Ciclos  WPROT") "Ciclos  WPROT"] -> w4794
          tunnel: w4791 -> [w4797 w4802]
          tunnel: [w4797 w4801] -> w4790
          tunnel: w4789 -> [w4796 w4800]
          tunnel: [w4796 w4799] -> w4788
          frame False {
          }
          frame True {
            n2361 = call-dynamic "Write Obs_state.vi"("error in (no error)"=w4800, "Obs_state"=u32 350, "S4ACS_GUI in"=w4802) -> ("error out"=w4799:errorcluster, "S4ACS_GUI out"=w4801:refnum<class "S4GUI.lvclass">)  [unwired: 7 in]
          }
        }
        n2362 = call-dynamic "Write cycles wprot.vi"("error in (no error)"=w4788, "cycles wprot"=w4794, "S4GUI in"=w4790) -> ("error out"=w4792:errorcluster, "S4GUI out"=w4793:refnum<class "S4GUI.lvclass">)  [unwired: 7 in]
      }
      event "Start SM": Value Change {
        n2363 = event-data() -> ()  [unwired: 1 in, 6 out]
        n2364 = call-dynamic "Read Obs_state.vi"("error in (no error)"=w4831, "S4ACS_GUI in"=w4832) -> ("error out"=w4818:errorcluster, "Obs_state"=w4829:u32, "S4ACS_GUI out"=w4820:refnum<class "S4GUI.lvclass">)  [unwired: 7 in]
        n2365 = call "Read Instrument.lvclass.vi"("error in (no error)"=w4818, "S4ACS_GUI in"=w4820) -> ("error out"=w4816:errorcluster, "Instrument.lvclass"=w4817:refnum<class "Instrument.lvclass">, "S4ACS_GUI out"=w4819:refnum<class "S4GUI.lvclass">)  [unwired: 7 in]
        n2366 = Not Equal?(x=w4829, y=u32 400) -> (x != y?=w4828:bool)
        n2367 = call-dynamic "Read mode.vi"("error in (no error)"=w4816, "Instrument in"=w4817) -> ("error out"=w4815:errorcluster, "mode"=w4814:bool)  [unwired: 7 in, 1 out]
        n2368 = case shown="True" w4828 {
          tunnel: w4819 -> [w4874 w4962]
          tunnel: w4815 -> [w4875 w4961]
          tunnel: [w4878 w4975] -> w4809
          tunnel: [w4877 w4973] -> w4808
          tunnel: w4825 -> [_ w4982]
          tunnel: w4824 -> [_ w4981]
          tunnel: w4823 -> [_ w4980]
          tunnel: w4822 -> [_ w4979]
          tunnel: w4821 -> [_ w4978]
          tunnel: w4814 -> [_ w4977]
          tunnel: w4813 -> [_ w4952]
          tunnel: w4812 -> [_ w4955]
          tunnel: w4811 -> [_ w4954]
          tunnel: w4810 -> [_ w4953]
          tunnel: ["RESUME SM CLICKED" ("User Event") "START SM" ("User Event")] -> w4805
          frame False {
            # "Obs_state=400 (PAUSED), envia RESUME e vai para Obs_state=500 \npara esperar envio do comando RESUME a todos os canais."
            n2369 = call-dynamic "Write Obs_state.vi"("error in (no error)"=w4875, "Obs_state"=500, "S4ACS_GUI in"=w4874) -> ("error out"=w4879:errorcluster, "S4ACS_GUI out"=w4880:refnum<class "S4GUI.lvclass">)  [unwired: 7 in]
            n2370 = call-dynamic "Read AcquisitionA.vi"("error in (no error)"=w4879, "S4ACS_GUI in"=w4880) -> ("error out"=w4866:errorcluster, "Acquisition.lvclass"=w4870:refnum<class "Acquisition.lvclass">, "S4ACS_GUI out"=w4890:refnum<class "S4GUI.lvclass">)  [unwired: 7 in]
            n2371 = call-dynamic "Read enabled.vi"("error in (no error)"=w4866, "Server in"=w4870) -> ("error out"=w4868:errorcluster, "enabled"=w4867:bool, "Server out"=w4869:refnum<class "Acquisition.lvclass">)  [unwired: 7 in]
            n2372 = call-dynamic "Read Channel.vi"("error in (no error)"=w4868, "Acquisition in"=w4869) -> ("error out"=w4871:errorcluster, "Channel.lvclass"=w4872:refnum<class "Channel.lvclass">, "Acquisition out"=w4889:refnum<class "Acquisition.lvclass">)  [unwired: 7 in]
            n2373 = case shown="True" w4867 {
              tunnel: w4889 -> [w4937 w4950]
              tunnel: [w4937 w4949] -> w4888
              tunnel: [w4936 w4946] -> w4887
              tunnel: w4872 -> [_ w4939]
              tunnel: w4871 -> [w4936 w4938]
              frame False {
              }
              frame True {
                n2374 = call-dynamic "Read State Machine.vi"("error in (no error)"=w4938, "Device in"=w4939) -> ("error out"=w4940:errorcluster, "State Machine.lvclass"=w4941:refnum<class "State Machine.lvclass">, "Device out"=w4945:refnum<class "Channel.lvclass">)  [unwired: 7 in]
                n2375 = call "Next State.vi"("error in (no error)"=w4940, "New_State"=96, "State Machine in"=w4941) -> ("error out"=w4942:errorcluster, "State Machine out"=w4944:refnum<class "State Machine.lvclass">)  [unwired: 7 in]
                n2376 = call-dynamic "Write State Machine.vi"("error in (no error)"=w4942, "State Machine.lvclass"=w4944, "Device in"=w4945) -> ("error out"=w4947:errorcluster, "Device out"=w4948:refnum<class "Channel.lvclass">)  [unwired: 7 in]
                n2377 = call-dynamic "Write Channel.vi"("error in (no error)"=w4947, "Channel.lvclass"=w4948, "Acquisition in"=w4950) -> ("error out"=w4946:errorcluster, "Acquisition out"=w4949:refnum<class "Acquisition.lvclass">)  [unwired: 7 in]
              }
            }
            n2378 = call-dynamic "Write AcquisitionA.vi"("error in (no error)"=w4887, "Acquisition.lvclass"=w4888, "S4ACS_GUI in"=w4890) -> ("error out"=w4886:errorcluster, "S4ACS_GUI out"=w4883:refnum<class "S4GUI.lvclass">)  [unwired: 7 in]
            n2379 = call "Read AcquisitionB.vi"("error in (no error)"=w4886, "S4ACS_GUI in"=w4883) -> ("error out"=w4857:errorcluster, "Acquisition.lvclass"=w4858:refnum<class "Acquisition.lvclass">, "S4ACS_GUI out"=w4859:refnum<class "S4GUI.lvclass">)  [unwired: 7 in]
            n2380 = call-dynamic "Read enabled.vi"("error in (no error)"=w4857, "Server in"=w4858) -> ("error out"=w4861:errorcluster, "enabled"=w4860:bool, "Server out"=w4862:refnum<class "Acquisition.lvclass">)  [unwired: 7 in]
            n2381 = call-dynamic "Read Channel.vi"("error in (no error)"=w4861, "Acquisition in"=w4862) -> ("error out"=w4863:errorcluster, "Channel.lvclass"=w4864:refnum<class "Channel.lvclass">, "Acquisition out"=w4865:refnum<class "Acquisition.lvclass">)  [unwired: 7 in]
            n2382 = case shown="True" w4860 {
              tunnel: w4865 -> [w4922 w4935]
              tunnel: [w4922 w4934] -> w4856
              tunnel: [w4921 w4931] -> w4855
              tunnel: w4864 -> [_ w4924]
              tunnel: w4863 -> [w4921 w4923]
              frame False {
              }
              frame True {
                n2383 = call-dynamic "Read State Machine.vi"("error in (no error)"=w4923, "Device in"=w4924) -> ("error out"=w4925:errorcluster, "State Machine.lvclass"=w4926:refnum<class "State Machine.lvclass">, "Device out"=w4930:refnum<class "Channel.lvclass">)  [unwired: 7 in]
                n2384 = call "Next State.vi"("error in (no error)"=w4925, "New_State"=96, "State Machine in"=w4926) -> ("error out"=w4927:errorcluster, "State Machine out"=w4929:refnum<class "State Machine.lvclass">)  [unwired: 7 in]
                n2385 = call-dynamic "Write State Machine.vi"("error in (no error)"=w4927, "State Machine.lvclass"=w4929, "Device in"=w4930) -> ("error out"=w4932:errorcluster, "Device out"=w4933:refnum<class "Channel.lvclass">)  [unwired: 7 in]
                n2386 = call-dynamic "Write Channel.vi"("error in (no error)"=w4932, "Channel.lvclass"=w4933, "Acquisition in"=w4935) -> ("error out"=w4931:errorcluster, "Acquisition out"=w4934:refnum<class "Acquisition.lvclass">)  [unwired: 7 in]
              }
            }
            n2387 = call "Write AcquisitionB.vi"("error in (no error)"=w4855, "Acquisition.lvclass"=w4856, "S4ACS_GUI in"=w4859) -> ("error out"=w4885:errorcluster, "S4ACS_GUI out"=w4882:refnum<class "S4GUI.lvclass">)  [unwired: 7 in]
            n2388 = call-dynamic "Read AcquisitionC.vi"("error in (no error)"=w4885, "S4ACS_GUI in"=w4882) -> ("error out"=w4845:errorcluster, "Acquisition.lvclass"=w4848:refnum<class "Acquisition.lvclass">, "S4ACS_GUI out"=w4847:refnum<class "S4GUI.lvclass">)  [unwired: 7 in]
            n2389 = call-dynamic "Read enabled.vi"("error in (no error)"=w4845, "Server in"=w4848) -> ("error out"=w4850:errorcluster, "enabled"=w4849:bool, "Server out"=w4851:refnum<class "Acquisition.lvclass">)  [unwired: 7 in]
            n2390 = call-dynamic "Read Channel.vi"("error in (no error)"=w4850, "Acquisition in"=w4851) -> ("error out"=w4852:errorcluster, "Channel.lvclass"=w4853:refnum<class "Channel.lvclass">, "Acquisition out"=w4854:refnum<class "Acquisition.lvclass">)  [unwired: 7 in]
            n2391 = case shown="True" w4849 {
              tunnel: w4854 -> [w4907 w4920]
              tunnel: [w4907 w4919] -> w4846
              tunnel: [w4906 w4916] -> w4844
              tunnel: w4853 -> [_ w4909]
              tunnel: w4852 -> [w4906 w4908]
              frame False {
              }
              frame True {
                n2392 = call-dynamic "Read State Machine.vi"("error in (no error)"=w4908, "Device in"=w4909) -> ("error out"=w4910:errorcluster, "State Machine.lvclass"=w4911:refnum<class "State Machine.lvclass">, "Device out"=w4915:refnum<class "Channel.lvclass">)  [unwired: 7 in]
                n2393 = call "Next State.vi"("error in (no error)"=w4910, "New_State"=96, "State Machine in"=w4911) -> ("error out"=w4912:errorcluster, "State Machine out"=w4914:refnum<class "State Machine.lvclass">)  [unwired: 7 in]
                n2394 = call-dynamic "Write State Machine.vi"("error in (no error)"=w4912, "State Machine.lvclass"=w4914, "Device in"=w4915) -> ("error out"=w4917:errorcluster, "Device out"=w4918:refnum<class "Channel.lvclass">)  [unwired: 7 in]
                n2395 = call-dynamic "Write Channel.vi"("error in (no error)"=w4917, "Channel.lvclass"=w4918, "Acquisition in"=w4920) -> ("error out"=w4916:errorcluster, "Acquisition out"=w4919:refnum<class "Acquisition.lvclass">)  [unwired: 7 in]
              }
            }
            n2396 = call-dynamic "Write AcquisitionC.vi"("error in (no error)"=w4844, "Acquisition.lvclass"=w4846, "S4ACS_GUI in"=w4847) -> ("error out"=w4884:errorcluster, "S4ACS_GUI out"=w4881:refnum<class "S4GUI.lvclass">)  [unwired: 7 in]
            n2397 = call-dynamic "Read AcquisitionD.vi"("error in (no error)"=w4884, "S4ACS_GUI in"=w4881) -> ("error out"=w4835:errorcluster, "Acquisition.lvclass"=w4836:refnum<class "Acquisition.lvclass">, "S4ACS_GUI out"=w4837:refnum<class "S4GUI.lvclass">)  [unwired: 7 in]
            n2398 = call-dynamic "Read enabled.vi"("error in (no error)"=w4835, "Server in"=w4836) -> ("error out"=w4839:errorcluster, "enabled"=w4838:bool, "Server out"=w4840:refnum<class "Acquisition.lvclass">)  [unwired: 7 in]
            n2399 = call-dynamic "Read Channel.vi"("error in (no error)"=w4839, "Acquisition in"=w4840) -> ("error out"=w4841:errorcluster, "Channel.lvclass"=w4842:refnum<class "Channel.lvclass">, "Acquisition out"=w4843:refnum<class "Acquisition.lvclass">)  [unwired: 7 in]
            n2400 = case shown="True" w4838 {
              tunnel: w4843 -> [w4892 w4905]
              tunnel: [w4892 w4904] -> w4834
              tunnel: [w4891 w4901] -> w4833
              tunnel: w4842 -> [_ w4894]
              tunnel: w4841 -> [w4891 w4893]
              frame False {
              }
              frame True {
                n2401 = call-dynamic "Read State Machine.vi"("error in (no error)"=w4893, "Device in"=w4894) -> ("error out"=w4895:errorcluster, "State Machine.lvclass"=w4896:refnum<class "State Machine.lvclass">, "Device out"=w4900:refnum<class "Channel.lvclass">)  [unwired: 7 in]
